vi "Execute.vi"(8 "error in (no error)":errorcluster, 10 "Context in":refnum<class "Context.lvclass">, 11 "Complete Manual Command in":refnum<class "Complete Manual Command.lvclass">) -> (0 "error out":errorcluster, 2 "Context out":refnum<class "Context.lvclass">, 3 "Complete Manual Command out":refnum<class "Complete Manual Command.lvclass">)   [LabVIEW 2016, in "Complete Manual Command.lvclass"]
uses:
  Complete Manual Command.lvclass
  Context/Context.lvclass
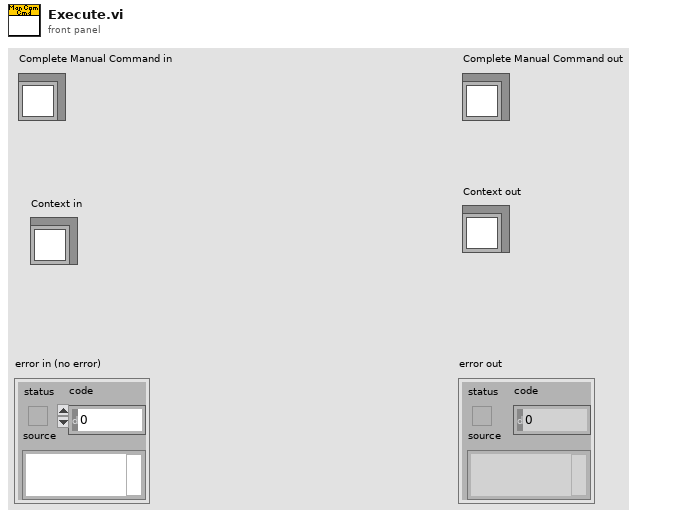
[diagram p1: front panel]
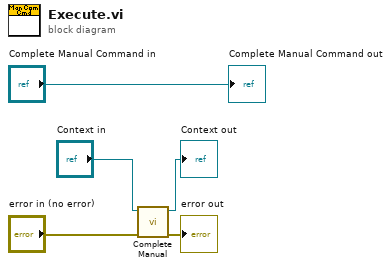
[diagram p0: block diagram]
diagram:
  n1 = call "Complete Manual.vi"("error in (no error)"="error in (no error)", "Context in"="Context in") -> ("error out"=→"error out":errorcluster, "Context out"=→"Context out":refnum<class "Context.lvclass">)  [unwired: 8 in]
  "Complete Manual Command out" <- "Complete Manual Command in"
